vi "ClassAttributes_ReadWriteClassAttributes_4x4x4_Singleton.vi"(8 "error in (no error)":errorcluster) -> (0 "error out":errorcluster)   [LabVIEW 2014]
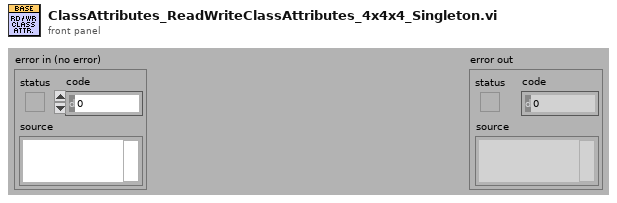
[diagram p1: front panel]
types:
  T1 = typedef "ClassAttributes_ClassAttributes.ctl" = cluster{"classAttribute1":bool}
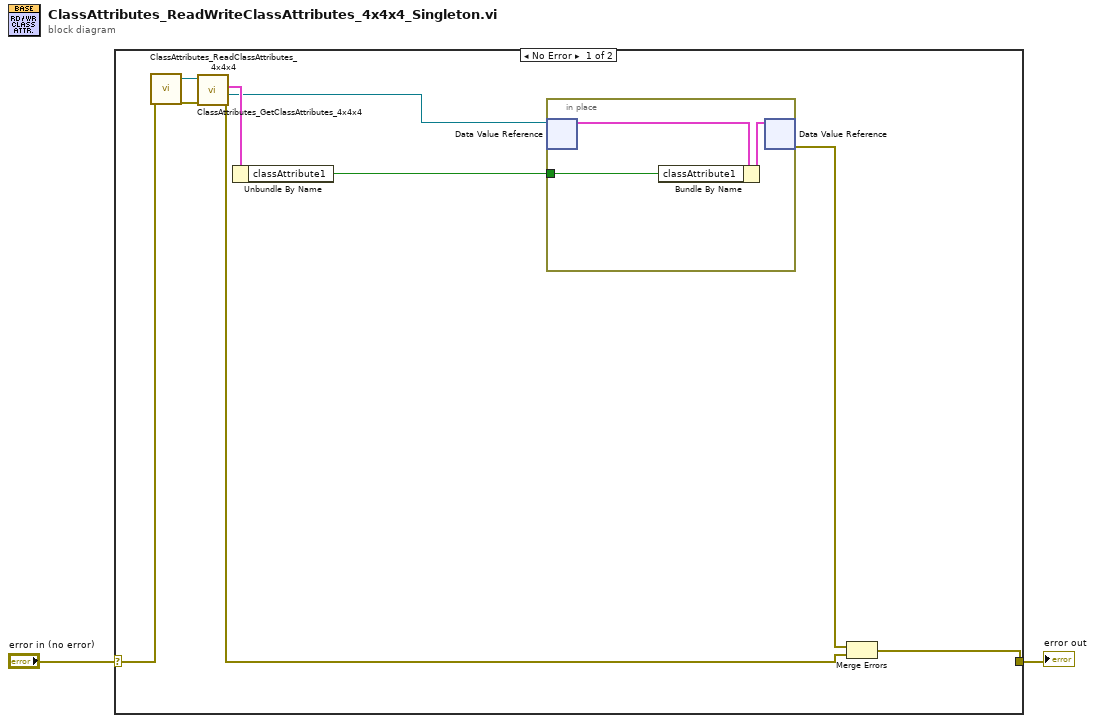
[diagram p0: block diagram]
diagram:
  n1 = case shown="No Error" "error in (no error)" {
    selector: "error in (no error)" -> [w3 w15]
    tunnel: [w6 w15] -> w1
    frame No Error {
      n2 = call <resource>:"ClassAttributes_ReadClassAttributes_4x4x4.vi"("error in (no error)"=w3) -> ("error out"=w4:errorcluster, "reference out"=w5:refnum<class>)  [unwired: 9 in]
      n3 = call <resource>:"ClassAttributes_GetClassAttributes_4x4x4.vi"("error in (no error)"=w4, "reference in"=w5) -> ("error out"=w7:errorcluster, "Class attribute Reference"=w9:refnum<data-value>, "Class attribute"=w11:T1)  [unwired: 6 in, 1 out]
      n4 = Unbundle By Name(w11) -> ("classAttribute1"=w8:bool)
      n5 = in-place {
        in-place-border: w8 -> [w14]
        n6 = in-place-dvr #1(w9) -> (w13:T1)  [unwired: 1 out]
        n7 = Bundle By Name(cluster=w13, "classAttribute1"=w14) -> (w12:T1)
        n8 = in-place-dvr #1(w12) -> (w10:errorcluster)  [unwired: 1 out]
      }
      n9 = Merge Errors(w10, w7) -> (w6:errorcluster)
    }
    frame Error {
    }
  }
  "error out" <- w1
